vi "FindAndAim.vi"(8 "error in":errorcluster, 11 "Speed/Direction":dbl) -> (0 "error out":errorcluster)   [LabVIEW 2016]
uses:
  Robot Global Data.vi
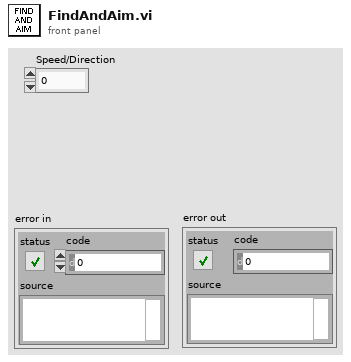
[diagram p1: front panel]
types:
  T1 = cluster{"Target?":bool, "Angle":dbl, "Distance":dbl}
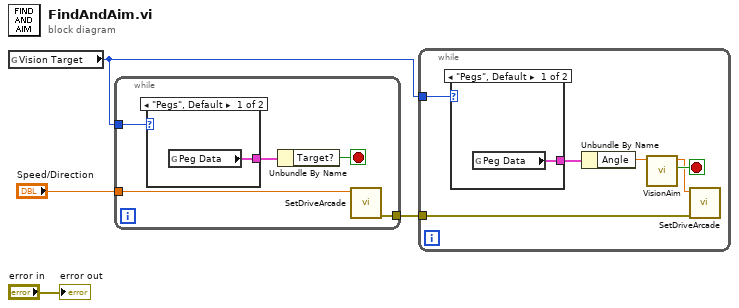
[diagram p0: block diagram]
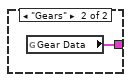
[diagram p2: hidden frame]
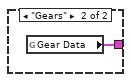
[diagram p3: hidden frame]
diagram:
  n1 = global read "Robot Global Data.vi" "Vision Target"() -> (w2:enum16{"Pegs", "Gears"})
  n2 = while {
    tunnel: w2 -> [w9]
    tunnel: "Speed/Direction" -> [w8]
    tunnel: [w5] -> w1
    stop <- w6 stop-if-true
    n3 = case shown="\"Pegs\", Default" w9 {
      tunnel: [w10 w11] -> w7
      frame "Pegs", Default {
        n4 = global read "Robot Global Data.vi" "Peg Data"() -> (w10:T1)
      }
      frame "Gears" {
        n5 = global read "Robot Global Data.vi" "Gear Data"() -> (w11:T1)
      }
    }
    n6 = Unbundle By Name(w7) -> ("Target?"=w6:bool)
    n7 = call "SetDriveArcade.vi"("Turn"=w8) -> ("error out"=w5:errorcluster)  [unwired: 10 in]
  }
  n8 = while {
    tunnel: w2 -> [w17]
    tunnel: w1 -> [w12]
    stop <- w16 stop-if-true
    n9 = case shown="\"Pegs\", Default" w17 {
      tunnel: [w18 w19] -> w15
      frame "Pegs", Default {
        n10 = global read "Robot Global Data.vi" "Peg Data"() -> (w18:T1)
      }
      frame "Gears" {
        n11 = global read "Robot Global Data.vi" "Gear Data"() -> (w19:T1)
      }
    }
    n12 = Unbundle By Name(w15) -> ("Angle"=w14:dbl)
    n13 = call "VisionAim.vi"("Angle"=w14) -> ("In Range"=w16:bool, "Turn"=w13:dbl)  [unwired: 9 in]
    n14 = call "SetDriveArcade.vi"("error in"=w12, "Turn"=w13) -> ()  [unwired: 9 in, 1 out]
  }
  "error out" <- "error in"
